vi "MasterKey.String.ConvertToChannelValues.vi"(11 "Master Key":string) -> (2 "Length":i32, 3 "Value":u64)   [LabVIEW 2019, in "Diagnostics Addon Shared.lvlib"]
uses:
  Diagnostics Addon Shared.lvlib
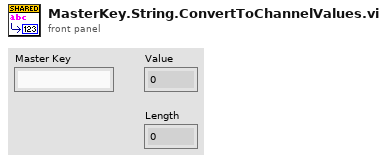
[diagram p1: front panel]
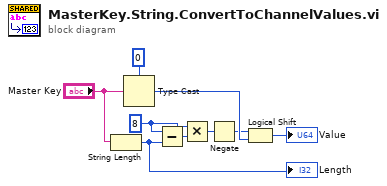
[diagram p0: block diagram]
diagram:
  w1 = 8 ("x")
  n1 = String Length(string="Master Key") -> (length=w2:i32)
  "Length" <- w2
  n2 = Type Cast(type=u64 0, x="Master Key") -> (*(type *) &x=w8:u64)
  n3 = Subtract(x=w1, y=w2) -> (x-y=w7:i32)
  n4 = Multiply(x=w1, y=w7) -> (x*y=w6:i32)
  n5 = Negate(x=w6) -> (-x=w5:i32)
  n6 = Logical Shift(y=w5, x=w8) -> (x << y=→"Value":u64)
